vi "Convert hex coordinate into decimal number.vi"(11 "Coordinate":string) -> (2 "Decimal number (not rounded)":dbl, 3 "Decimal number (rounded)":i32)   [LabVIEW 2010]
panel:
  # "000A0300"
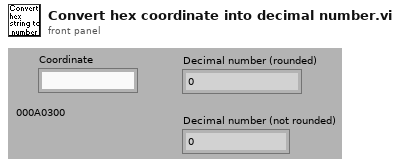
[diagram p1: front panel]
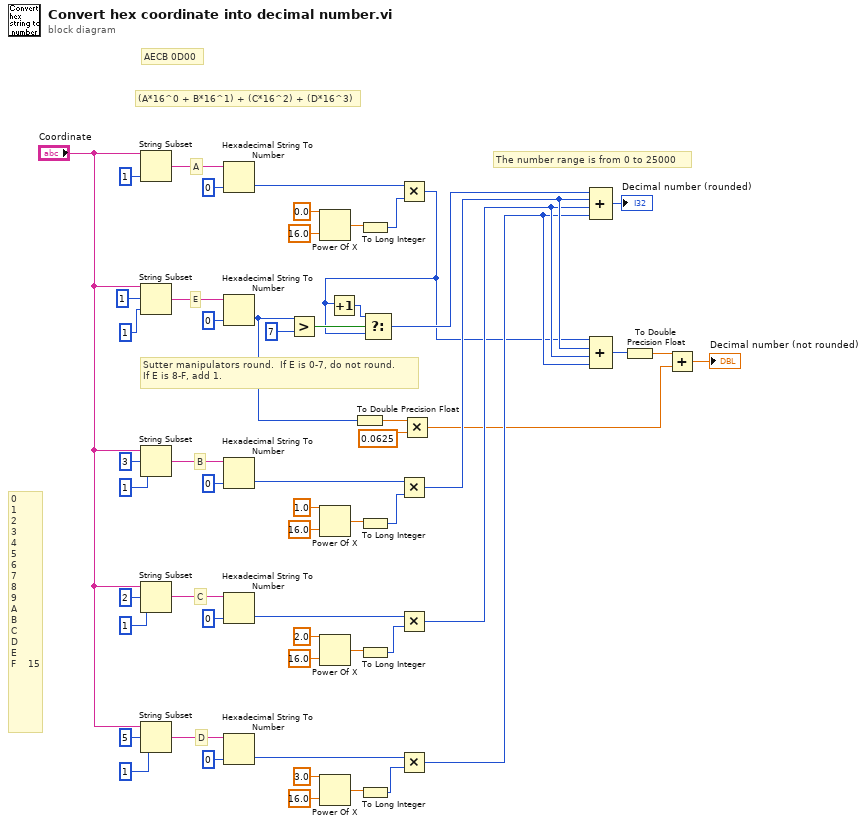
[diagram p0: block diagram]
diagram:
  # "0    \n1\n2\n3\n4\n5\n6\n7\n8\n9\nA\nB\nC\nD\nE\nF    15"
  # "The number range is from 0 to 25000"
  # "Sutter manipulators round.  If E is 0-7, do not round.\nIf E is 8-F, add 1."
  # "E"
  # "D"
  # "B"
  # "C"
  # "A"
  # "(A*16^0 + B*16^1) + (C*16^2) + (D*16^3)"
  # "AECB 0D00"
  n1 = String Subset(string="Coordinate", length (rest)=1 ("length (rest)")) -> (substring=w47:string)  [unwired: 1 out]
  n2 = String Subset(string="Coordinate", offset (0)=1, length (rest)=1 ("length (rest)")) -> (substring=w19:string)
  n3 = String Subset(string="Coordinate", offset (0)=3, length (rest)=1 ("length (rest)")) -> (substring=w37:string)
  n4 = String Subset(string="Coordinate", offset (0)=2, length (rest)=1 ("length (rest)")) -> (substring=w34:string)
  n5 = String Subset(string="Coordinate", offset (0)=5, length (rest)=1 ("length (rest)")) -> (substring=w33:string)
  n6 = Hexadecimal String To Number(string=w47, default (0uL)=0 ("default (0 U32)")) -> (number=w46:i32)  [unwired: 2 out]
  n7 = Hexadecimal String To Number(string=w19, default (0uL)=0 ("default (0 U32)")) -> (number=w7:i32)  [unwired: 2 out]
  n8 = Hexadecimal String To Number(string=w37, default (0uL)=0 ("default (0 U32)")) -> (number=w39:i32)  [unwired: 2 out]
  n9 = Hexadecimal String To Number(string=w34, default (0uL)=0 ("default (0 U32)")) -> (number=w32:i32)  [unwired: 2 out]
  n10 = Hexadecimal String To Number(string=w33, default (0uL)=0 ("default (0 U32)")) -> (number=w31:i32)  [unwired: 2 out]
  n11 = Greater?(x=w7, y=7) -> (0:w14:bool)
  n12 = Power Of X(1:16.0 ("x"), 2:0.0 ("y")) -> (0:w45:dbl)
  n13 = Power Of X(1:16.0 ("x"), 2:1.0 ("y")) -> (0:w40:dbl)
  n14 = Power Of X(1:16.0 ("x"), 2:2.0 ("y")) -> (0:w26:dbl)
  n15 = Power Of X(1:16.0 ("x"), 2:3.0 ("y")) -> (0:w24:dbl)
  n16 = To Double Precision Float(number=w7) -> (double precision float=w6:dbl)
  n17 = To Long Integer(number=w45) -> (32bit integer=w44:i32)
  n18 = To Long Integer(number=w40) -> (32bit integer=w41:i32)
  n19 = To Long Integer(number=w26) -> (32bit integer=w25:i32)
  n20 = To Long Integer(number=w24) -> (32bit integer=w21:i32)
  n21 = Multiply(x=w46, y=w44) -> (x*y=w8:i32)
  n22 = Increment(x=w8) -> (x+1=w13:i32)
  n23 = Select(t=w13, s=w14, f=w8) -> (s? t:f=w12:i32)
  n24 = Multiply(x=w39, y=w41) -> (x*y=w11:i32)
  n25 = Multiply(x=w32, y=w25) -> (x*y=w10:i32)
  n26 = Multiply(x=w31, y=w21) -> (x*y=w9:i32)
  n27 = Multiply(x=w6, y=0.0625) -> (x*y=w2:dbl)
  n28 = Compound Arithmetic op=ADD(w12, w11, w10, w9) -> (→"Decimal number (rounded)":i32)
  n29 = Compound Arithmetic op=ADD(w8, w11, w10, w9) -> (w4:i32)
  n30 = To Double Precision Float(number=w4) -> (double precision float=w3:dbl)
  n31 = Add(x=w3, y=w2) -> (x+y=→"Decimal number (not rounded)":dbl)
